vi "_Publish DP Indicators(Refmgr).vi"(7 "VIRef(Caller VI)":T1, 8 "error in (no error)":errorcluster, 9 "force update(F)":bool, 11 "SILAPI In":T1) -> (0 "error out":errorcluster, 1 "Binded DPs":string[](array[string]), 3 "SILAPI Out":T1)   [LabVIEW 2017, in "TagDB RefManager.lvlib"]
uses:
  TagDB RefManager.lvlib
  <userlib>/_NEVSTOP/TagDB/Typedef/TagDB.ctl
  10d0bc68-ff5b-4b3e-94b6-72122e87f5c0.vi
  9ac63a17-9284-407c-a5c8-8910fcebbfe1.vi
  99199be5-3273-4500-92d5-279e96ad7927.vi
  0f9c47dc-4cad-44a4-9ff9-6b222f0d776a.vi
  <userlib>/_NEVSTOP/TagDB/_Support/DataAccess/_NameCacher.vi
  <userlib>/_NEVSTOP/TagDB/_Support/Error/_[error50002]Invalid DataType.vi
  <userlib>/_NEVSTOP/TagDB/_Support/Error/_[error50000]Invalid DB REF.vi
  <userlib>/_NEVSTOP/TagDB/_Support/DataAccess/TagDB Ref to DVR.vi
  <userlib>/_NEVSTOP/TagDB/_Support/URL/TRIM-BOTH-SPACE.vi
  9ac63a17-9284-407c-a5c8-8910fcebbfe1.vi/1b47866c-8e2d-43a7-815f-8cf18635e5a1.vi
  0f9c47dc-4cad-44a4-9ff9-6b222f0d776a.vi/1b47866c-8e2d-43a7-815f-8cf18635e5a1.vi
  <userlib>/_NEVSTOP/TagDB/_Support/Change Detector/TagDB dbChanged.vi
  <userlib>/_NEVSTOP/TagDB/_Support/Error/_Clear Errors.vi
  9ac63a17-9284-407c-a5c8-8910fcebbfe1.vi/1b47866c-8e2d-43a7-815f-8cf18635e5a1.vi/29b2ea6d-6d7f-4e4a-ad31-a5cb760462c7.vi
  <userlib>/_NEVSTOP/TagDB/API/TagDB-Status.vi
  0f9c47dc-4cad-44a4-9ff9-6b222f0d776a.vi/1b47866c-8e2d-43a7-815f-8cf18635e5a1.vi/29b2ea6d-6d7f-4e4a-ad31-a5cb760462c7.vi
  <userlib>/_NEVSTOP/TagDB/_Support/Change Detector/TagDB ChangeFlag.vi
  <userlib>/_NEVSTOP/TagDB/_Support/Error/_Build Error Cluster.vi
  <userlib>/_NEVSTOP/TagDB/TagDB.lvlib
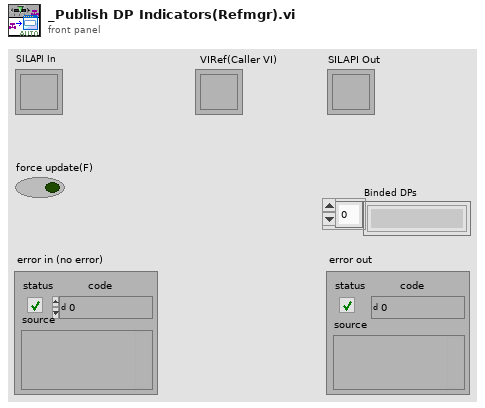
[diagram p1: front panel]
types:
  T1 = typedef "TagDB.lvlib/TagDB.ctl" = refnum<k1>
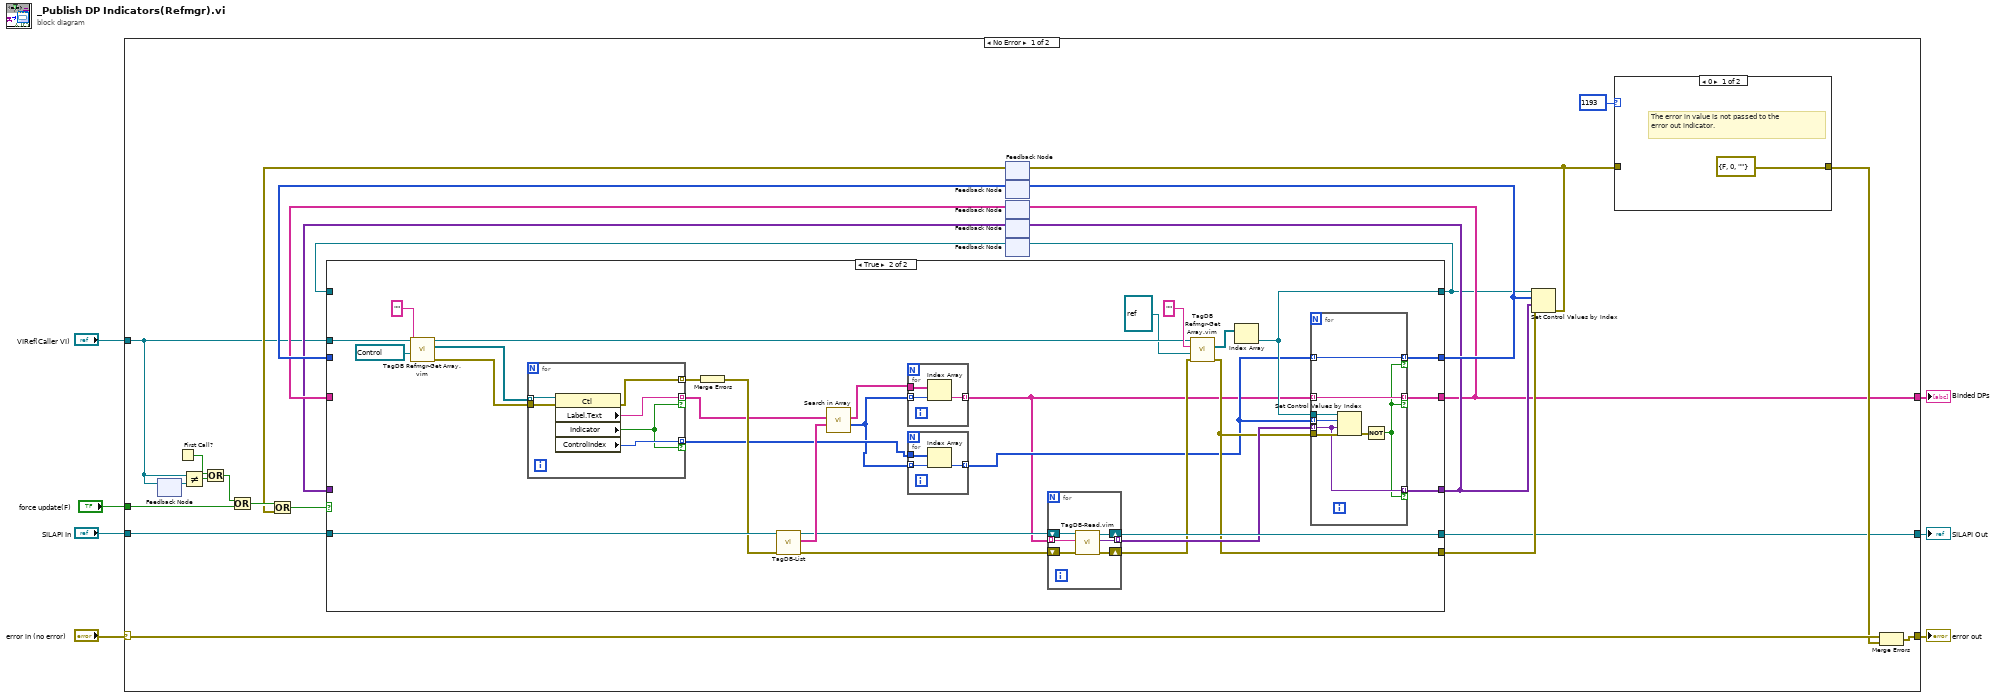
[diagram p0: block diagram]
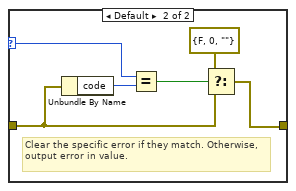
[diagram p2: hidden frame]
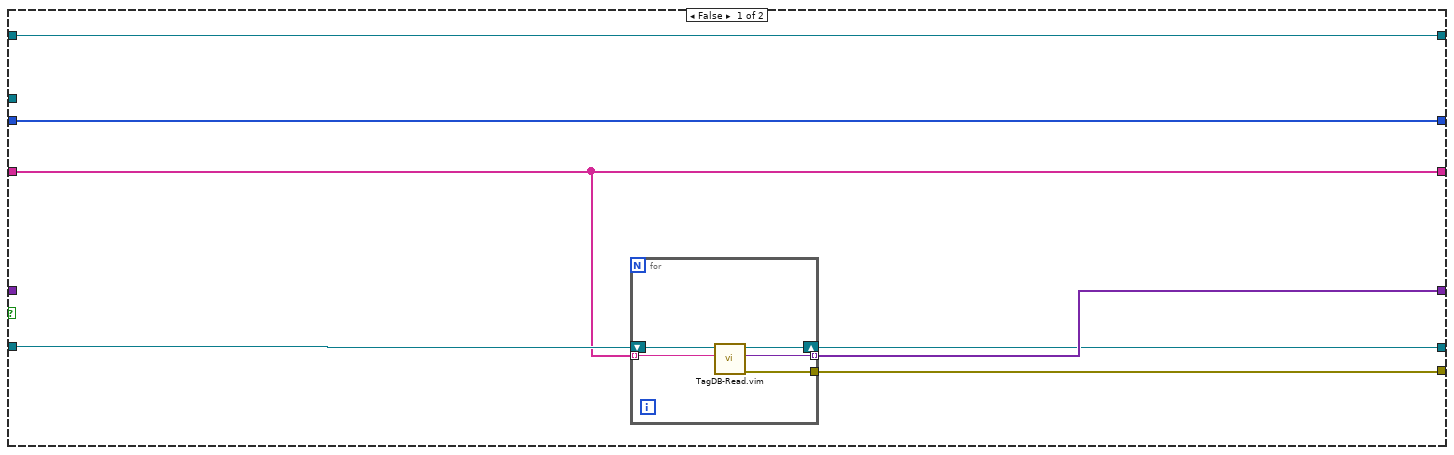
[diagram p3: hidden frame]
diagram:
  n1 = case shown="No Error" "error in (no error)" {
    selector: "error in (no error)" -> [w27 w107]
    tunnel: "force update(F)" -> [w32 _]
    tunnel: [w28 w107] -> w6
    tunnel: "SILAPI In" -> [w25 w108]
    tunnel: [w20 _] -> w3
    tunnel: "VIRef(Caller VI)" -> [w11 _]
    tunnel: [w15 w108] -> w1
    frame No Error {
      n2 = feedback-in #1(w11) -> ()
      n3 = feedback #1() -> (w12:T1)  [unwired: 1 in]
      n4 = First Call?() -> (First Call?: T/F=w9:bool)
      n5 = Not Equal?(x=w11, y=w12) -> (x != y?=w10:bool)
      n6 = Or(x=w9, y=w10) -> (x .or. y?=w8:bool)
      n7 = Or(x=w8, y=w32) -> (x .or. y?=w29:bool)
      n8 = feedback #2() -> (w17:errorcluster)  [unwired: 1 in]
      n9 = Or(x=w29, y=w17) -> (x .or. y?=w19:bool)
      n10 = feedback #3() -> (w30:i32[])  [unwired: 1 in]
      n11 = feedback #4() -> (w26:string[])  [unwired: 1 in]
      n12 = feedback #5() -> (w22:variant[])  [unwired: 1 in]
      n13 = feedback #6() -> (w13:refnum<vi>)  [unwired: 1 in]
      n14 = case shown="True" w19 {
        tunnel: [w40 w58] -> w14
        tunnel: w11 -> [_ w80]
        tunnel: [w46 w74] -> w31
        tunnel: w30 -> [w46 _]
        tunnel: [w44 w75] -> w20
        tunnel: w26 -> [w44 _]
        tunnel: [w42 w73] -> w23
        tunnel: w25 -> [w45 w79]
        tunnel: [w43 w59] -> w24
        tunnel: w22 -> [_ _]
        tunnel: [w41 w77] -> w15
        tunnel: w13 -> [w40 _]
        frame False {
          n15 = for {
            tunnel: w44 -> [w50] mode=indexing
            tunnel: [w49] -> w43
            tunnel: [w48] -> w42 mode=indexing
            shift-right: [w47] -> w41
            shift-left: w45 -> [w51]
            n16 = call "TagDB-Read.vim"("name"=w50, "TagDB"=w51) -> ("error out"=w49:errorcluster, "Value"=w48:variant, "TagDB(dup)"=w47:T1)  [unwired: 4 in, 3 out]
          }
        }
        frame True {
          n17 = call "TagDB Refmgr-Get Array.vim"("Type"=refnum<vi> refnum, "RegExp"="", "DB Ref"=w80) -> ("error out"=w66:errorcluster, "References"=w65:refnum<vi>[], "DB Ref(dup)"=w63:T1)  [unwired: 5 in, 1 out]
          n18 = for {
            tunnel: w65 -> [w98] mode=indexing
            tunnel: [w97] -> w53 mode=indexing if=w95
            tunnel: [w96] -> w56 mode=indexing if=w95
            tunnel: [w94] -> w72 mode=indexing
            tunnel: w66 -> [w93]
            n19 = property class="Ctl"(reference=w98, error in=w93) -> (error out=w94:errorcluster, "Label.Text"=w97:string, "Indicator"=w95:bool, "ControlIndex"=w96:i32)  [unwired: 1 out]
          }
          n20 = Merge Errors(w72) -> (w71:errorcluster)
          n21 = call <userlib>:"TagDB-List.vi"("error in (no error)"=w71, "TagDB"=w79) -> ("error out"=w78:errorcluster, "names"=w70:string[], "TagDB(dup)"=w69:T1)  [unwired: 6 in, 1 out]
          n22 = call "Search in Array.vi"("items to filter"=w70, "array"=w53) -> ("item Indexs"=w54:i32[], "array(dup)"=w52:string[])  [unwired: 4 in]
          n23 = for {
            tunnel: w54 -> [w83] mode=indexing
            tunnel: w52 -> [w82]
            tunnel: [w81] -> w55 mode=indexing
            n24 = Index Array(array=w82, index=w83) -> (element=w81:string)
          }
          n25 = for {
            tunnel: w54 -> [w86] mode=indexing
            tunnel: w56 -> [w85]
            tunnel: [w84] -> w57 mode=indexing
            n26 = Index Array(array=w85, index=w86) -> (element=w84:i32)
          }
          n27 = for {
            tunnel: [w90] -> w76 mode=indexing
            tunnel: w55 -> [w88] mode=indexing
            shift-right: [w89] -> w60
            shift-left: w78 -> [w92]
            shift-right: [w91] -> w77
            shift-left: w69 -> [w87]
            n28 = call "TagDB-Read.vim"("error in (no error)"=w92, "name"=w88, "TagDB"=w87) -> ("error out"=w89:errorcluster, "Value"=w90:variant, "TagDB(dup)"=w91:T1)  [unwired: 3 in, 3 out]
          }
          n29 = call "TagDB Refmgr-Get Array.vim"("error in (no error)"=w60, "Type"=refnum<vi> refnum ("Current VI Reference"), "RegExp"="", "DB Ref"=w63) -> ("error out"=w59:errorcluster, "References"=w61:refnum<vi>[])  [unwired: 4 in, 2 out]
          n30 = Index Array(array=w61) -> (element=w58:refnum<vi>)  [unwired: 1 in]
          n31 = for {
            tunnel: w58 -> [w106]
            tunnel: w57 -> [w105] mode=indexing
            tunnel: w76 -> [w101] mode=indexing
            tunnel: w59 -> [w104]
            tunnel: [w103] -> w75 mode=indexing if=w99
            tunnel: w55 -> [w103] mode=indexing
            tunnel: [w102] -> w74 mode=indexing if=w99
            tunnel: w57 -> [w102] mode=indexing
            tunnel: [w101] -> w73 mode=indexing if=w99
            n32 = Set Control Values by Index(0:w106, 1:w105, 2:w101, 3:w104) -> (11:w100:errorcluster)
            n33 = Not(x=w100) -> (.not. x?=w99:bool)
          }
        }
      }
      n34 = feedback-in #3(w31) -> ()
      n35 = feedback-in #4(w20) -> ()
      n36 = feedback-in #5(w23) -> ()
      n37 = feedback-in #6(w14) -> ()
      n38 = Set Control Values by Index(0:w14, 1:w31, 2:w23, 3:w24) -> (11:w18:errorcluster)
      n39 = feedback-in #2(w18) -> ()
      n40 = case shown="0" 1193 ("specific error code to clear (0: all)") {
        selector: 1193 ("specific error code to clear (0: all)") -> [_ w38]
        tunnel: w18 -> [_ w37]
        tunnel: [errorcluster {"status"=FALSE, "code"=0, "source"=""} ("error constant") w34] -> w21
        frame 0 {
          # "The error in value is not passed to the\nerror out indicator."
        }
        frame Default {
          # "Clear the specific error if they match. Otherwise, output error in value."
          n41 = Unbundle By Name(w37) -> ("code"=w39:i32)
          n42 = Equal?(x=w38, y=w39) -> (x = y?=w35:bool)
          n43 = Select(t=errorcluster {"status"=FALSE, "code"=0, "source"=""} ("error constant"), s=w35, f=w37) -> (s? t:f=w34:errorcluster)
        }
      }
      n44 = Merge Errors(w27, w21) -> (w28:errorcluster)
    }
    frame Error {
    }
  }
  "error out" <- w6
  "SILAPI Out" <- w1
  "Binded DPs" <- w3
